vi "testCheckQueueToDdsFull.vi"(8 "error in (no error)":errorcluster) -> (0 "error out":errorcluster)   [LabVIEW 2018]
doc: "Test the checkQueueFull.vi with queueToDds option."
uses:
  src/TcpServer/TcpServer.lvclass
  src/TcpServerTel/typedef/queueOptionsTypeDef.ctl
  src/TcpServerTel/typedef/enqueueOptionsTypeDef.ctl
  src/TcpServer/TcpServer.lvclass/TcpServer.ctl
  src/TcpServerTel/typedef/telTypeDef.ctl
  src/TcpServerBase/TcpServerBase.lvclass/TcpServerBase.ctl
  src/TcpServerTel/TcpServerTel.lvclass
  home/pcortes/github/ts_labview_tcp_json/src/TcpServerBase/TcpServerBase.lvclass
  <vilib>/addons/_JKI Toolkits/Caraya/classes/Assert/Assert False.vi
  <vilib>/addons/_JKI Toolkits/Caraya/classes/Assert/Assert True.vi
  <vilib>/addons/_JKI Toolkits/Caraya/classes/Test/Test.lvclass
  <vilib>/addons/_JKI Toolkits/Caraya/classes/Assert/Assert.lvclass
  src/TcpServerBase/TcpServerBase.lvclass
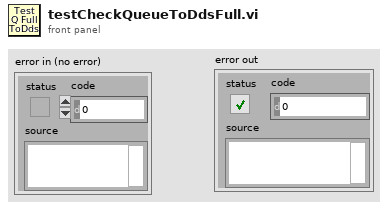
[diagram p1: front panel]
types:
  T1 = typedef "TcpServerTel.lvclass/enqueueOptionsTypeDef.ctl" = enum16{"lossy enqueue", "normal enqueue"}
  T2 = cluster{"cmdServerPort":u16, "telServerPort":u16, "serverTimeout (ms)":i32, "serverBytesToRead":i32, "maxSizeQueueTel":i32, "EnqueueOptions":T1, "timeoutQueueTel (ms)":i32, "tcpClientQueueMaxSize":i32, "timeoutInMs":i32}
  T3 = typedef "TcpServerTel.lvclass/queueOptionsTypeDef.ctl" = cluster{"EnqueueOptions":T1, "Timeout (ms)":i32}
  T4 = typedef "TcpServerTel.lvclass/telTypeDef.ctl" = cluster{"name":string, "telDetails":string}
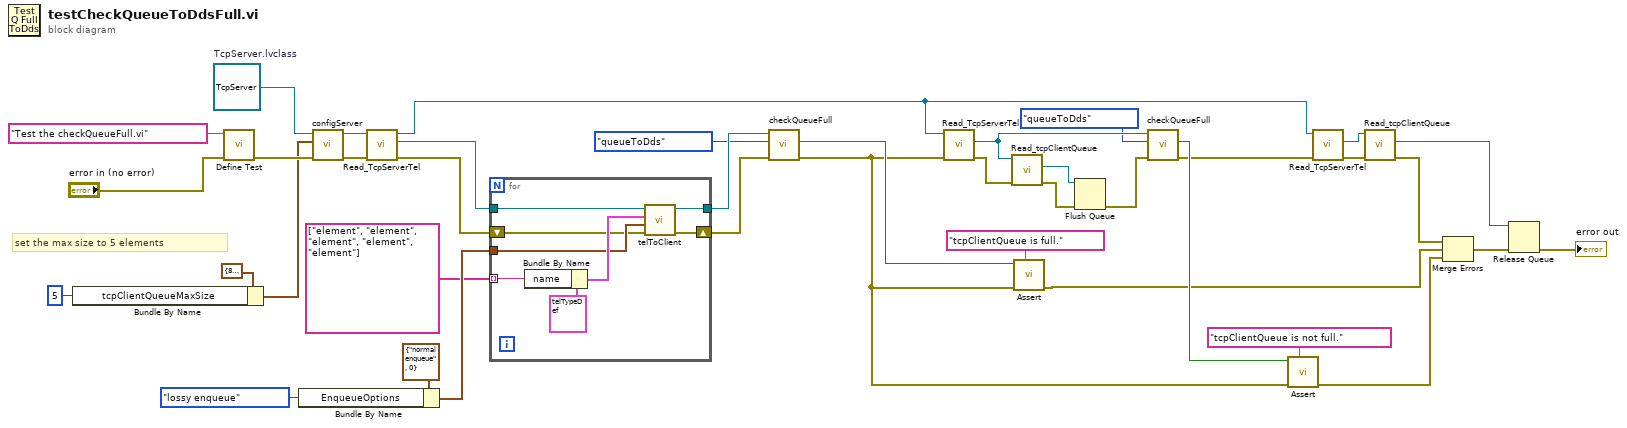
[diagram p0: block diagram]
diagram:
  w28 = refnum<class "TcpServer.lvclass"> refnum  # TcpServer.lvclass
  # "set the max size to 5 elements"
  n1 = Bundle By Name(cluster=T2 {"cmdServerPort"=8888, "telServerPort"=8889, "serverTimeout (ms)"=100, "serverBytesToRead"=32768, "maxSizeQueueTel"=1000, "EnqueueOptions"=enum."lossy enqueue", "timeoutQueueTel (ms)"=50, "tcpClientQueueMaxSize"=1000, "timeoutInMs"=100} ("ServerConfiguration"), "tcpClientQueueMaxSize"=5 ("telQueueServerMaxSize")) -> (w2:T2)
  n2 = call <vilib>:"Define Test.vi"("error in (no error)"="error in (no error)", "Label (VI Title)"="Test the checkQueueFull.vi") -> ("error out"=w27:errorcluster)  [unwired: 9 in]
  n3 = Bundle By Name(cluster=T3 {"EnqueueOptions"=enum."normal enqueue", "Timeout (ms)"=0} ("queueOptions"), "EnqueueOptions"=enqueueOptionsTypeDef."lossy enqueue") -> (w20:T3)
  n4 = call "configServer.vi"("error in (no error)"=w27, "ServerConfiguration"=w2, "tcpServer in"=w28) -> ("error out"=w25:errorcluster, "tcpServer out"=w26:refnum<class "TcpServer.lvclass">)  [unwired: 7 in]
  n5 = call "Read_TcpServerTel.vi"("error in (no error)"=w25, "TcpServer in"=w26) -> ("error out"=w23:errorcluster, "TcpServerTel.lvclass"=w24:refnum<class "TcpServerTel.lvclass">, "TcpServer out"=w5:refnum<class "TcpServer.lvclass">)  [unwired: 7 in]
  n6 = for {
    tunnel: w24 -> [w47]
    tunnel: w20 -> [w43]
    shift-right: [w41] -> w19
    shift-left: w23 -> [w42]
    tunnel: string[] ["element", "element", "element", "element", "element"] -> [w45] mode=indexing
    tunnel: [w40] -> w7
    n7 = Bundle By Name(cluster=T4 {"name"="elevation", "telDetails"="\"compName\":\"MTMount\""} ("Telemetry"), "name"=w45) -> (w44:T4)
    n8 = call "telToClient.vi"("error in (no error)"=w42, "queueOptions"=w43, "Telemetry"=w44, "TcpServerTel in"=w47) -> ("error out"=w41:errorcluster, "TcpServerTel out"=w40:refnum<class "TcpServerTel.lvclass">)  [unwired: 6 in]
  }
  n9 = call "checkQueueFull.vi"("error in (no error)"=w19, "queueName"=enum16{"queueFromDds", "queueToDds"}."queueToDds", "tcpServerTel in"=w7) -> ("error out"=w13:errorcluster, "queueFull"=w34:bool)  [unwired: 6 in, 1 out]
  n10 = call "Read_TcpServerTel.vi"("error in (no error)"=w13, "TcpServer in"=w5) -> ("error out"=w18:errorcluster, "TcpServerTel.lvclass"=w6:refnum<class "TcpServerTel.lvclass">)  [unwired: 7 in, 1 out]
  n11 = call "Read_tcpClientQueue.vi"("error in (no error)"=w18, "TcpServerBase in"=w6) -> ("error out"=w16:errorcluster, "tcpClientQueue"=w17:refnum<queue>)  [unwired: 7 in, 1 out]
  n12 = call-poly <vilib>:"Assert.vi"("Label"="tcpClientQueue is full.", "error in (no error)"=w13, "True?"=w34) -> ("error out"=w10:errorcluster)  [unwired: 8 in]
  n13 = Flush Queue(queue=w17, error in (no error)=w16) -> (error out=w15:errorcluster)  [unwired: 2 out]
  n14 = call "checkQueueFull.vi"("error in (no error)"=w15, "queueName"=enum16{"queueFromDds", "queueToDds"}."queueToDds", "tcpServerTel in"=w6) -> ("error out"=w11:errorcluster, "queueFull"=w12:bool)  [unwired: 6 in, 1 out]
  n15 = call-poly <vilib>:"Assert.vi"("Label"="tcpClientQueue is not full.", "error in (no error)"=w13, "False?"=w12) -> ("error out"=w9:errorcluster)  [unwired: 8 in]
  n16 = call "Read_TcpServerTel.vi"("error in (no error)"=w11, "TcpServer in"=w5) -> ("error out"=w33:errorcluster, "TcpServerTel.lvclass"=w32:refnum<class "TcpServerTel.lvclass">)  [unwired: 7 in, 1 out]
  n17 = call "Read_tcpClientQueue.vi"("error in (no error)"=w33, "TcpServerBase in"=w32) -> ("error out"=w30:errorcluster, "tcpClientQueue"=w31:refnum<queue>)  [unwired: 7 in, 1 out]
  n18 = Merge Errors(w30, w10, w9) -> (w35:errorcluster)
  n19 = Release Queue(queue=w31, error in (no error)=w35) -> (error out=→"error out":errorcluster)  [unwired: 1 in, 2 out]
